vi "select roi.vi"(10 "Elements Selected":string[][](table), 11 "Spectrum":cluster{"Channels":dbl[], "Intensity":dbl[]}[](graph)) -> (3 "ROI Array":T1[](array[typedef]))   [LabVIEW 2023]
uses:
  control/ROI element.ctl
  <vilib>/Analysis/1siggen.llb/Ramp Pattern by Samples.vi
  <vilib>/Analysis/NI_AAL_SigProc.lvlib
  <vilib>/Analysis/NI_AALBase.lvlib
  <vilib>/Analysis/NI_AALPro.lvlib
panel:
  out "size(s) 2":i32
  out "size(s)":i32
  out "Locations":dbl[][](array[numeric])
  out "XY Graph":cluster{"Locations":dbl[], "Amplitudes":dbl[]}[](graph)
  in  "Parameters Fitted":dbl[][](array[numeric])
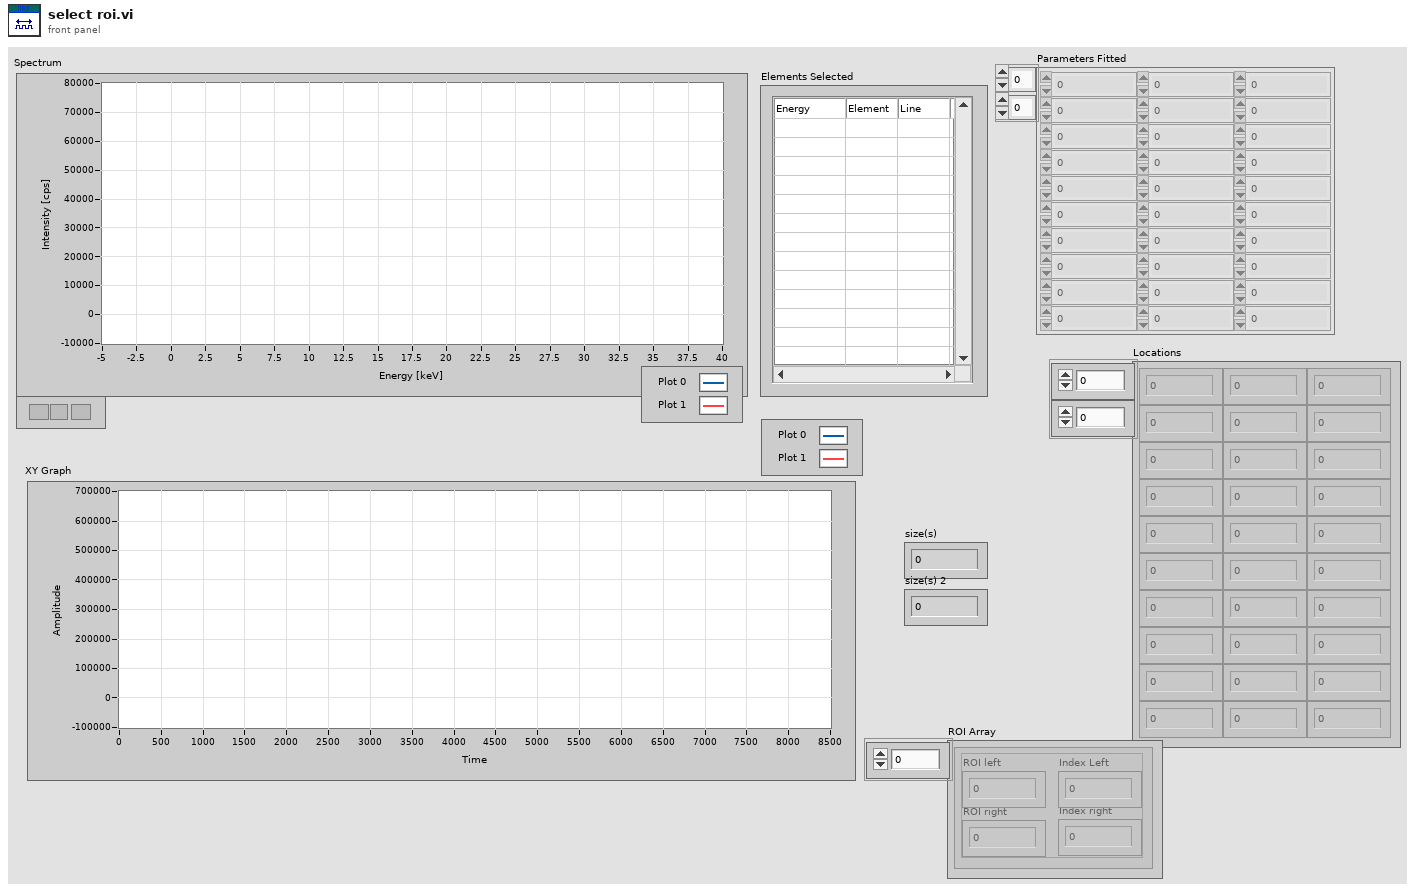
[diagram p1: front panel]
types:
  T1 = typedef "ROI element.ctl" = cluster{"ROI left":dbl, "Index Left":i32, "ROI right":dbl, "Index right":i32}
  T2 = cluster{"Ramp Pattern":dbl[], "Intensity":dbl[]}[]
  T3 = cluster{"initial amplitude":dbl, "initial center":dbl, "initial standard deviation":dbl, "offset":dbl}
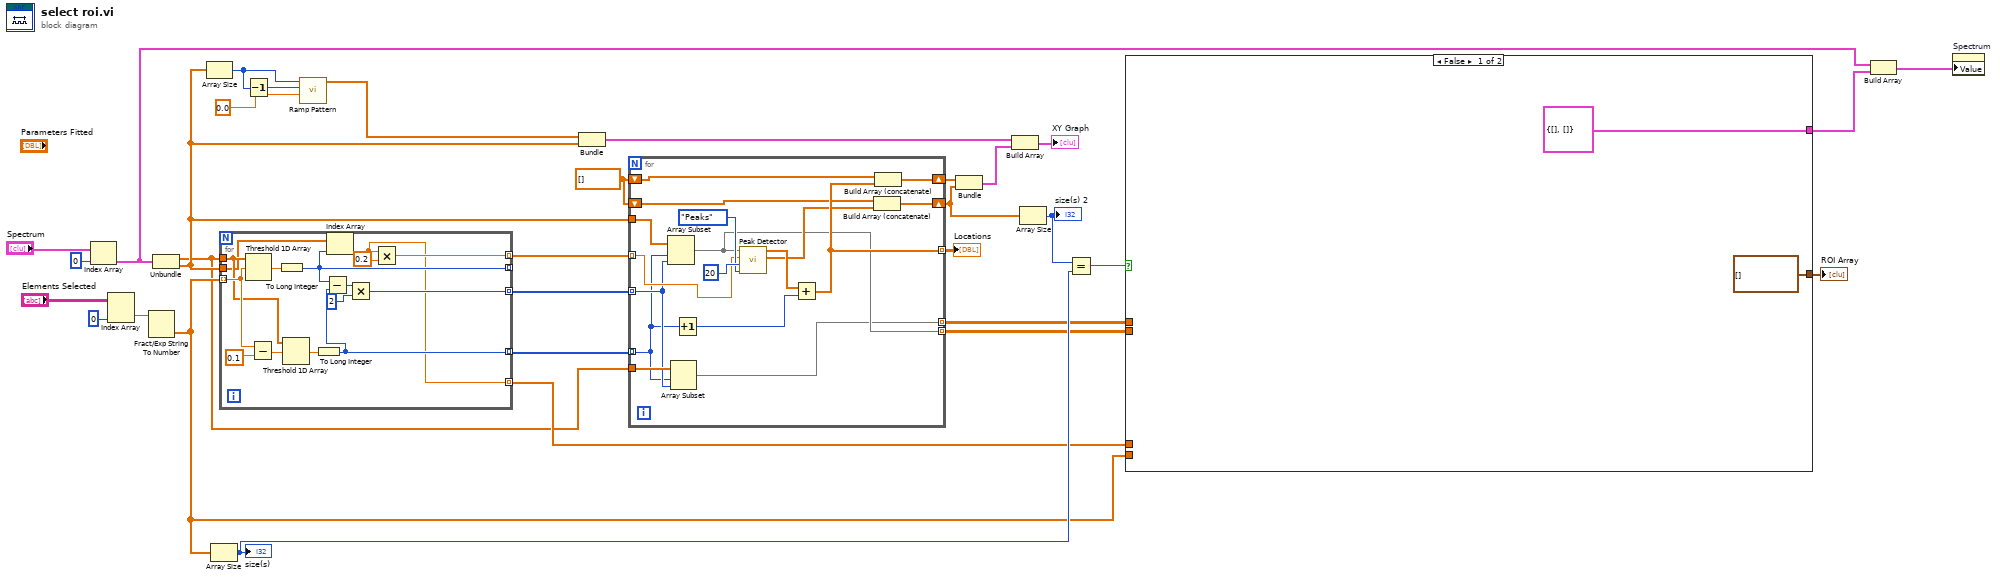
[diagram p0: block diagram]
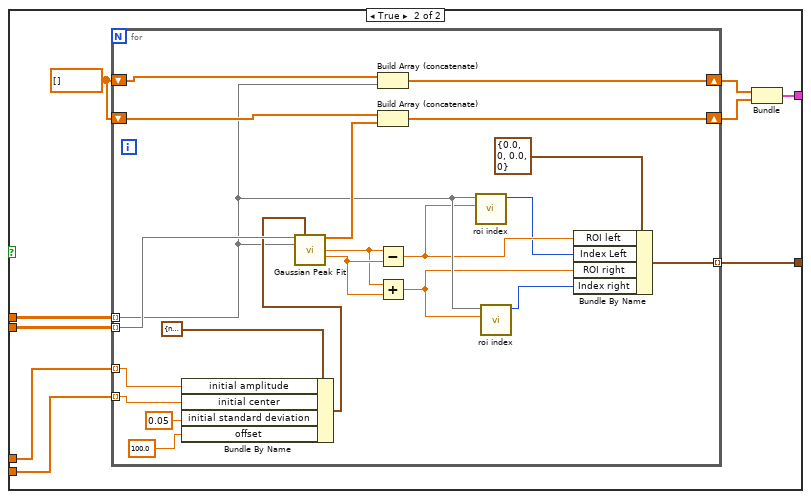
[diagram p2: hidden frame]
diagram:
  w17 = dbl[] []
  n1 = Index Array(array="Spectrum", index=0) -> (element=w4:cluster{"Channels":dbl[], "Intensity":dbl[]})
  n2 = Index Array(array="Elements Selected", index (col)=0 ("disabled index (col)")) -> (element=w30:string[])  [unwired: 1 in]
  n3 = Fract/Exp String To Number(string=w30) -> (number=w10:dbl[])  [unwired: 3 in, 1 out]
  n4 = Unbundle(w4) -> ("Channels"=w6:dbl[], "Intensity"=w18:dbl[])
  n5 = Array Size(array=w18) -> (size(s)=w23:i32)
  n6 = Array Size(array=w10) -> (size(s)=w12:i32)
  "size(s)" <- w12
  n7 = for {
    tunnel: w6 -> [w42]
    tunnel: w18 -> [w36]
    tunnel: w10 -> [w45] mode=indexing
    tunnel: [w37] -> _ mode=indexing
    tunnel: [w41] -> w27 mode=indexing
    tunnel: [w39] -> w26 mode=indexing
    tunnel: [w34] -> w8 mode=indexing
    tunnel: [w33] -> w7 mode=indexing
    n8 = Threshold 1D Array(2:w45, 3:w42) -> (0:w47:dbl)  [unwired: 1 in]
    n9 = Subtract(x=w45, y=0.1) -> (x-y=w43:dbl)
    n10 = To Long Integer(number=w47) -> (32bit integer=w37:i32)
    n11 = Threshold 1D Array(2:w43, 3:w42) -> (0:w44:dbl)  [unwired: 1 in]
    n12 = To Long Integer(number=w44) -> (32bit integer=w41:i32)
    n13 = Subtract(x=w37, y=w41) -> (x-y=w38:i32)
    n14 = Index Array(array=w36, index=w37) -> (element=w33:dbl)
    n15 = Multiply(x=w38, y=2) -> (x*y=w39:i32)
    n16 = Multiply(x=w33, y=0.2) -> (x*y=w34:dbl)
  }
  n17 = Decrement(x=w23) -> (x-1=w24:i32)
  n18 = call-poly <vilib>:"Ramp Pattern.vi"("start"=0.0, "end"=w24, "samples"=w23) -> ("Ramp Pattern"=w22:dbl[])  [unwired: 7 in, 1 out]
  n19 = Bundle("Ramp Pattern"=w22, "Intensity"=w18) -> (w21:cluster{"Ramp Pattern":dbl[], "Intensity":dbl[]})  [unwired: 1 in]
  n20 = for {
    tunnel: w18 -> [w64]
    tunnel: w27 -> [w49] mode=indexing
    tunnel: w26 -> [w50] mode=indexing
    tunnel: w8 -> [w53] mode=indexing
    tunnel: [w59] -> w19 mode=indexing
    shift-right: [w58] -> w16
    shift-left: w17 -> [w57]
    shift-right: [w56] -> w14
    shift-left: w17 -> [w54]
    tunnel: [w52] -> w9 mode=indexing
    tunnel: w6 -> [w51]
    tunnel: [w48] -> w5 mode=indexing
    n21 = Array Subset(array=w64, index=w49, length=w50) -> (w52:dbl[])
    n22 = Array Subset(array=w51, index=w49, length=w50) -> (w48:dbl[])
    n23 = Increment(x=w49) -> (x+1=w61:i32)
    n24 = call <vilib>:"Peak Detector.vi"("peaks/valleys"=enum32{"Peaks", "Valleys"}."Peaks", "width"=20, "threshold"=w53, "X"=w52) -> ("Amplitudes"=w55:dbl[], "Locations"=w60:dbl[])  [unwired: 3 in, 3 out]
    n25 = Add(x=w60, y=w61) -> (x+y=w59:dbl[])
    n26 = Build Array (concatenate)(w54, w55) -> (w56:dbl[])
    n27 = Build Array (concatenate)(w57, w59) -> (w58:dbl[])
  }
  "Locations" <- w19
  n28 = Bundle(w16, w14) -> (w15:cluster{dbl[], dbl[]})  [unwired: 1 in]
  n29 = Build Array(w21, w15) -> (→"XY Graph":T2)
  n30 = Array Size(array=w14) -> (size(s)=w13:i32)
  "size(s) 2" <- w13
  n31 = Equal?(x=w13, y=w12) -> (x = y?=w11:bool)
  n32 = case shown="False" w11 {
    tunnel: w10 -> [_ w73]
    tunnel: w9 -> [_ w75]
    tunnel: w7 -> [_ w74]
    tunnel: w5 -> [_ w72]
    tunnel: [cluster{dbl[], dbl[]} {[], []} w68] -> w3
    tunnel: [T1[] [] w67] -> w1
    frame False {
    }
    frame True {
      w71 = dbl[] []
      n33 = for {
        tunnel: w75 -> [w96] mode=indexing
        tunnel: w74 -> [w91] mode=indexing
        tunnel: w73 -> [w92] mode=indexing
        tunnel: w72 -> [w82] mode=indexing
        shift-right: [w88] -> w69
        shift-left: w71 -> [w85]
        shift-right: [w87] -> w70
        shift-left: w71 -> [w86]
        tunnel: [w76] -> w67 mode=indexing
        n34 = Bundle By Name(cluster=T3 {"initial amplitude"=nan, "initial center"=nan, "initial standard deviation"=nan, "offset"=nan} ("initial guess"), "initial amplitude"=w91, "initial center"=w92, "initial standard deviation"=0.05, "offset"=100.0) -> (w90:T3)
        n35 = call <vilib>:"Gaussian Peak Fit.vi"("Y"=w96, "initial guess"=w90, "X"=w82) -> ("Best Gaussian Fit"=w89:dbl[], "center"=w83:dbl, "standard deviation"=w84:dbl)  [unwired: 6 in, 4 out]
        n36 = Build Array (concatenate)(w86, w82) -> (w87:dbl[])
        n37 = Build Array (concatenate)(w85, w89) -> (w88:dbl[])
        n38 = Subtract(x=w83, y=w84) -> (x-y=w80:dbl)
        n39 = Add(x=w83, y=w84) -> (x+y=w78:dbl)
        n40 = call "roi index.vi"("Value"=w80, "Data"=w82) -> ("Minimum Element"=w79:i32)  [unwired: 9 in]
        n41 = call "roi index.vi"("Value"=w78, "Data"=w82) -> ("Minimum Element"=w77:i32)  [unwired: 9 in]
        n42 = Bundle By Name(cluster=T1 {"ROI left"=0.0, "Index Left"=0, "ROI right"=0.0, "Index right"=0} ("ROI element"), "ROI left"=w80, "Index Left"=w79, "ROI right"=w78, "Index right"=w77) -> (w76:T1)
      }
      n43 = Bundle(w70, w69) -> (w68:cluster{dbl[], dbl[]})  [unwired: 1 in]
    }
  }
  "ROI Array" <- w1
  n44 = Build Array(w4, w3) -> (w2:cluster{"Channels":dbl[], "Intensity":dbl[]}[])
  n45 = property on="Spectrum" class="XYGraph (strict)"("Value"=w2) -> ()  [unwired: 2 in, 2 out]
